vi "54-plate position.vi"(2 "position":T1={"X(A1)"=115.0, "Y(A1)"=125.0, "X(F9) "=218.0, "Y(F9) "=60.0, "count X"=9, "count Y"=6}) -> (5 "delta X":dbl, 6 "Array X":dbl[](array[numeric]), 7 "total":i32, 8 "delta Y":dbl, 9 "Array Y":dbl[](array[numeric]))   [LabVIEW 2023]
uses:
  Shared variables/position1.vi
  Shared variables/Shared variables.lvlib
panel:
  out "position1":dbl[][](array[numeric])
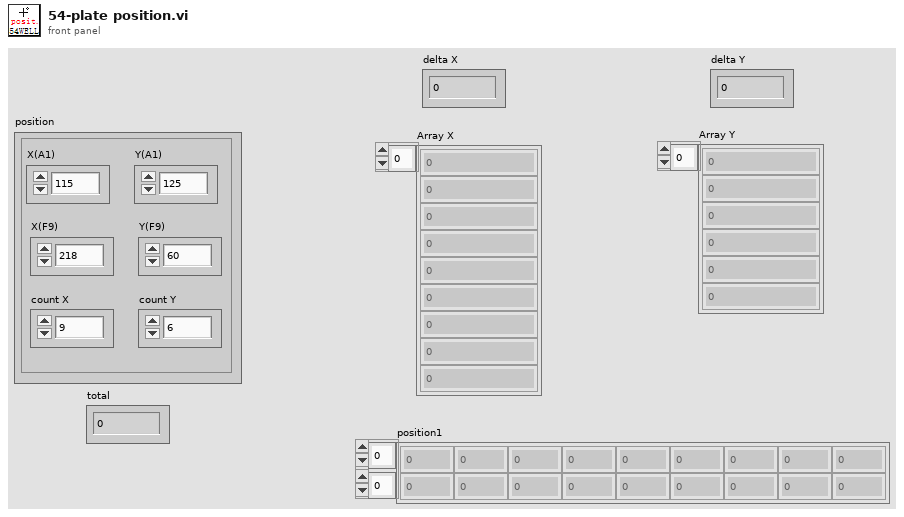
[diagram p1: front panel]
types:
  T1 = cluster{"X(A1)":dbl, "Y(A1)":dbl, "X(F9) ":dbl, "Y(F9) ":dbl, "count X":i32, "count Y":i32}
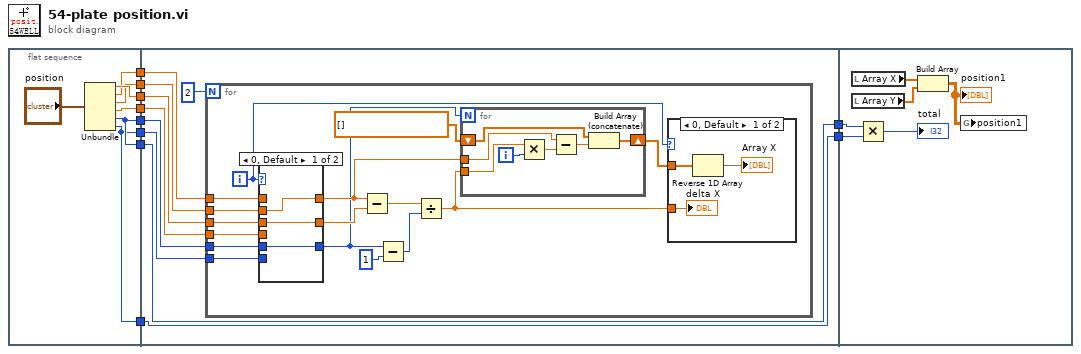
[diagram p0: block diagram]
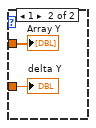
[diagram p2: hidden frame]
diagram:
  n1 = flat-sequence {
    tunnel: [w16] -> w10
    tunnel: [w15] -> w9
    tunnel: [w14] -> w8
    tunnel: [w13] -> w7
    tunnel: [w12] -> w6
    tunnel: [w11] -> w5
    tunnel: [w12] -> w3
    tunnel: [w11] -> w1
    tunnel: w10 -> [w25]
    tunnel: w9 -> [w24]
    tunnel: w8 -> [w23]
    tunnel: w7 -> [w22]
    tunnel: w6 -> [w21]
    tunnel: w5 -> [w20]
    tunnel: [w19] -> w4
    tunnel: w3 -> [w19]
    tunnel: [w18] -> w2
    tunnel: w1 -> [w18]
    tunnel: w4 -> [w65]
    tunnel: w2 -> [w64]
    frame #0 {
      n2 = Unbundle("position") -> ("X(A1)"=w16:dbl, "Y(A1)"=w15:dbl, "X(F9)"=w14:dbl, "Y(F9)"=w13:dbl, "count X"=w12:i32, "count Y"=w11:i32)
    }
    frame #1 {
      n3 = for {
        N: 2 -> [_]
        tunnel: w25 -> [w32]
        tunnel: w24 -> [w31]
        tunnel: w23 -> [w30]
        tunnel: w22 -> [w29]
        tunnel: w21 -> [w28]
        tunnel: w20 -> [w27]
        i -> [w34]
        n4 = case shown="0, Default" w34 {
          tunnel: w31 -> [_ w53]
          tunnel: w29 -> [_ w52]
          tunnel: w32 -> [w49 _]
          tunnel: w30 -> [w50 _]
          tunnel: [w50 w53] -> w36
          tunnel: [w49 w52] -> w35
          tunnel: [w48 w51] -> w33
          tunnel: w27 -> [_ w51]
          tunnel: w28 -> [w48 _]
          frame 0, Default {
          }
          frame 1 {
          }
        }
        n5 = Subtract(x=w36, y=w35) -> (x-y=w39:dbl)
        n6 = Subtract(x=w33, y=1) -> (x-y=w37:i32)
        n7 = Divide(x=w39, y=w37) -> (x/y=w42:dbl)
        n8 = for {
          N: w33 -> [_]
          shift-right: [w54] -> w41
          shift-left: dbl[] [] -> [w60]
          tunnel: w36 -> [w59]
          tunnel: w42 -> [w57]
          i -> [w58]
          n9 = Multiply(x=w57, y=w58) -> (x*y=w56:dbl)
          n10 = Subtract(x=w59, y=w56) -> (x-y=w55:dbl)
          n11 = Build Array (concatenate)(w60, w55) -> (w54:dbl[])
        }
        n12 = case shown="0, Default" w34 {
          tunnel: w42 -> [w45 w47]
          tunnel: w41 -> [w44 w46]
          frame 0, Default {
            n13 = Reverse 1D Array(array=w44) -> (reversed array=→"Array X":dbl[])
            "delta X" <- w45
          }
          frame 1 {
            "delta Y" <- w47
            "Array Y" <- w46
          }
        }
      }
    }
    frame #2 {
      n14 = local read "Array X"() -> (w63:dbl[])
      n15 = local read "Array Y"() -> (w62:dbl[])
      n16 = Multiply(x=w65, y=w64) -> (x*y=→"total":i32)
      n17 = Build Array(w63, w62) -> (w61:dbl[][])
      "position1" <- w61
      n18 = global write "position1.vi" "position1"(w61) -> ()
    }
  }
